vi "Data_Acquisition.vi"(5 "start Datetime":cluster{"row":i32, "column":i32}={"row"=1, "column"=0}, 7 "end Datetime":cluster{"row":i32, "column":i32}={"row"=3504, "column"=0}, 9 "start Data":cluster{"start row":i32, "start column":i32}={"start row"=1, "start column"=1}, 11 "end Data":cluster{"row":i32, "column":i32}={"row"=3504, "column"=4}) -> (8 "Meas":T1)   [LabVIEW 2022 SP3]
uses:
  <vilib>/Utility/NIReport.llb/Report Type.ctl
  <vilib>/addons/_office/excel.llb/Excel Get Data ([str]).vi
  <vilib>/addons/_office/excel.llb/Excel Get Data ([dbl]).vi
  <vilib>/Utility/NIReport.llb/NI_report.lvclass
  <vilib>/addons/_office/NI_ReportGenerationToolkit.lvlib
  <vilib>/Utility/NIReport.llb/NI_ReportGenerationCore.lvlib
  <vilib>/Utility/NIReport.llb/Excel/NI_Excel.lvclass
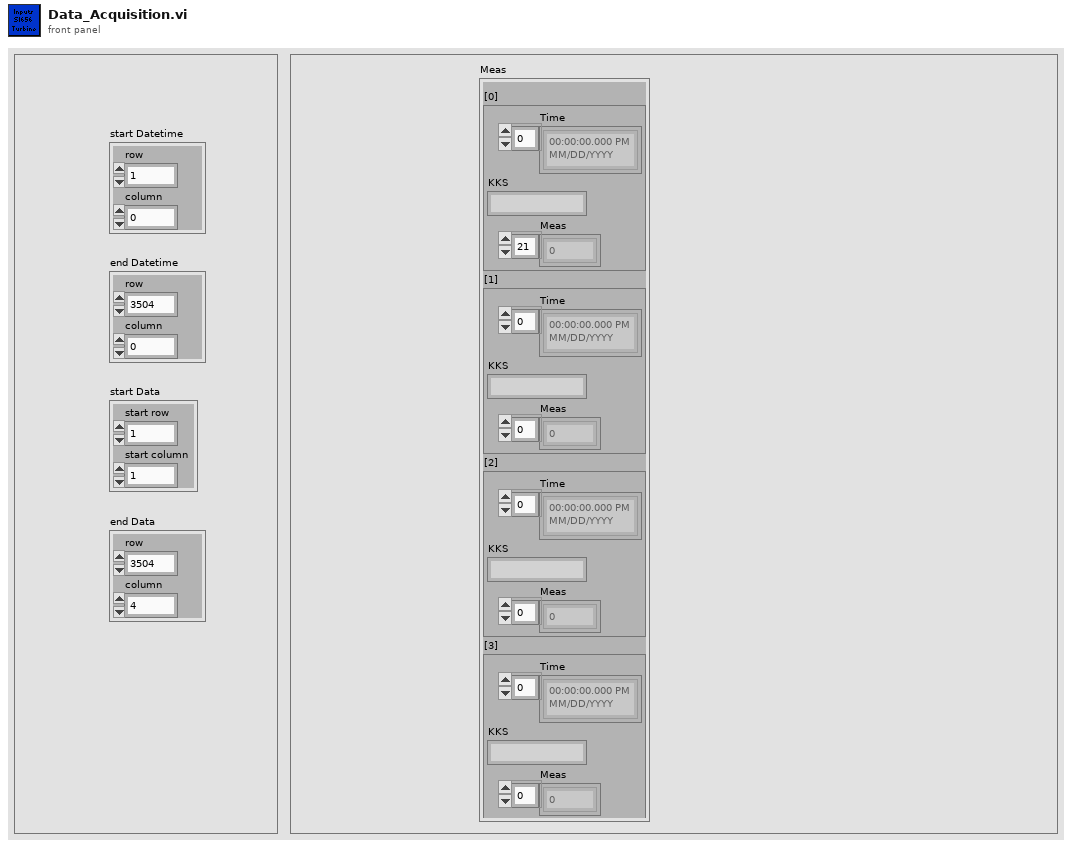
[diagram p1: front panel]
types:
  T1 = cluster{"[0]":cluster{"Time":timestamp[], "KKS":string, "Meas":dbl[]}, "[1]":cluster{"Time":timestamp[], "KKS":string, "Meas":dbl[]}, "[2]":cluster{"Time":timestamp[], "KKS":string, "Meas":dbl[]}, "[3]":cluster{"Time":timestamp[], "KKS":string, "Meas":dbl[]}, "[4]":cluster{"Time":timestamp[], "KKS":string, "Meas":dbl[]}, "[5]":cluster{"Time":timestamp[], "KKS":string, "Meas":dbl[]}, "[6]":cluster{"Time":timestamp[], "KKS":string, "Meas":dbl[]}, "[7]":cluster{"Time":timestamp[], "KKS":string, "Meas":dbl[]}, "[8]":cluster{"Time":timestamp[], "KKS":string, "Meas":dbl[]}}
  T2 = cluster{"Time":timestamp[], "KKS":string, "Meas":dbl[]}
  T3 = cluster{"Time":timestamp[], "KKS":string, "Meas":dbl[]}[]
  T4 = typedef "NI_ReportGenerationCore.lvlib/Report Type.ctl" = enum16{"HTML", "Word", "Excel"}
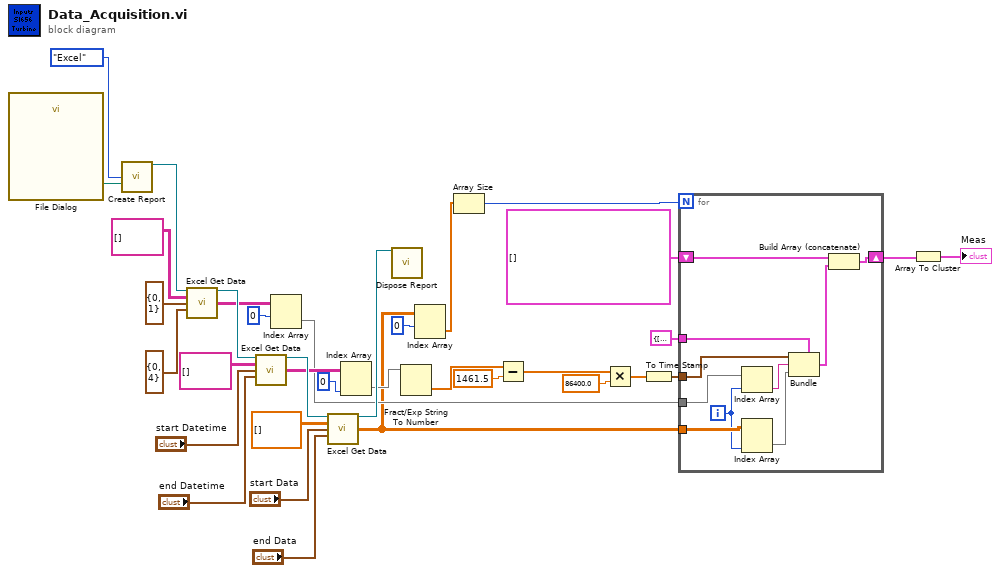
[diagram p0: block diagram]
diagram:
  n1 = call "File Dialog"() -> ("selected path"=w30:path)  [unwired: 12 in, 3 out]
  n2 = call <vilib>:"Create Report.vi"("report type"=Report_Type."Excel", "template (empty)"=w30) -> ("report out"=w17:refnum<class "NI_report.lvclass">)  [unwired: 12 in, 1 out]
  n3 = call-poly <vilib>:"Excel Get Data.vi"("report in"=w17, "data type"=string[][] [], "start (-1, -1)"=cluster{"start row":i32, "start column":i32} {"start row"=0, "start column"=1} ("start (0, 0)"), "end (-1, -1)"=cluster{"row":i32, "column":i32} {"row"=0, "column"=4}) -> ("report out"=w16:refnum<class "NI_report.lvclass">, "data"=w10:string[][])  [unwired: 9 in, 1 out]
  n4 = call-poly <vilib>:"Excel Get Data.vi"("report in"=w16, "data type"=string[][] [], "start (-1, -1)"="start Datetime", "end (-1, -1)"="end Datetime") -> ("report out"=w26:refnum<class "NI_report.lvclass">, "data"=w20:string[][])  [unwired: 9 in, 1 out]
  n5 = Index Array(array=w10, index (row)=0) -> (element=w8:string[])  [unwired: 1 in]
  n6 = call-poly <vilib>:"Excel Get Data.vi"("report in"=w26, "data type"=dbl[][] [], "start (-1, -1)"="start Data", "end (-1, -1)"="end Data") -> ("report out"=w32:refnum<class "NI_report.lvclass">, "data"=w6:dbl[][])  [unwired: 9 in, 1 out]
  n7 = Index Array(array=w20, index (col)=0 ("disabled index (col)")) -> (element=w18:string[])  [unwired: 1 in]
  n8 = call-dynamic "Dispose Report.vi"("report in"=w32) -> ()  [unwired: 14 in, 1 out]
  n9 = Fract/Exp String To Number(string=w18) -> (number=w25:dbl[])  [unwired: 3 in, 1 out]
  n10 = Index Array(array=w6, index (row)=0) -> (element=w4:dbl[])  [unwired: 1 in]
  n11 = Array Size(array=w4) -> (size(s)=w3:i32)
  n12 = Subtract(x=w25, y=1461.5) -> (x-y=w23:dbl[])
  n13 = Multiply(x=w23, y=86400.0) -> (x*y=w21:dbl[])
  n14 = To Time Stamp(1:w21) -> (0:w12:timestamp[])
  n15 = for {
    N: w3 -> [_]
    tunnel: w8 -> [w45]
    tunnel: w6 -> [w38]
    tunnel: w12 -> [w40]
    shift-right: [w42] -> w2
    shift-left: T3 [] -> [w41]
    tunnel: T2 {"Time"=[], "KKS"="", "Meas"=[]} -> [w39]
    i -> [w36]
    n16 = Index Array(array=w45, index=w36) -> (element=w44:string)
    n17 = Index Array(array=w38, index (col)=w36) -> (element=w37:dbl[])  [unwired: 1 in]
    n18 = Bundle(cluster=w39, "Time"=w40, "KKS"=w44, "Meas"=w37) -> (w43:T2)
    n19 = Build Array (concatenate)(w41, w43) -> (w42:T3)
  }
  n20 = Array To Cluster(array=w2) -> (cluster=→"Meas":T1)
